vi "atk_def.vi"(9 "IA State":T6, 10 "balls":T7[](array[typedef]), 11 "Robot in":T1) -> (3 "Robot out":T1)   [LabVIEW 2018]
uses:
  Core/AI Robot.ctl
  Functions Enum.ctl
  AttackerStates.ctl
  Path Planning/RRT/PathDests.ctl
  Path Planning/RRT/PathDest.ctl
  Core/AI Ball.ctl
  Core/AI Input.ctl
  Core/Field Size.ctl
  Core/AI Judge.ctl
  Command Enum.ctl
  Util/Events/Events.ctl
  <vilib>/Analysis/_algsub.llb/Real Vector Norm.vi
  <vilib>/Analysis/NI_AALPro.lvlib
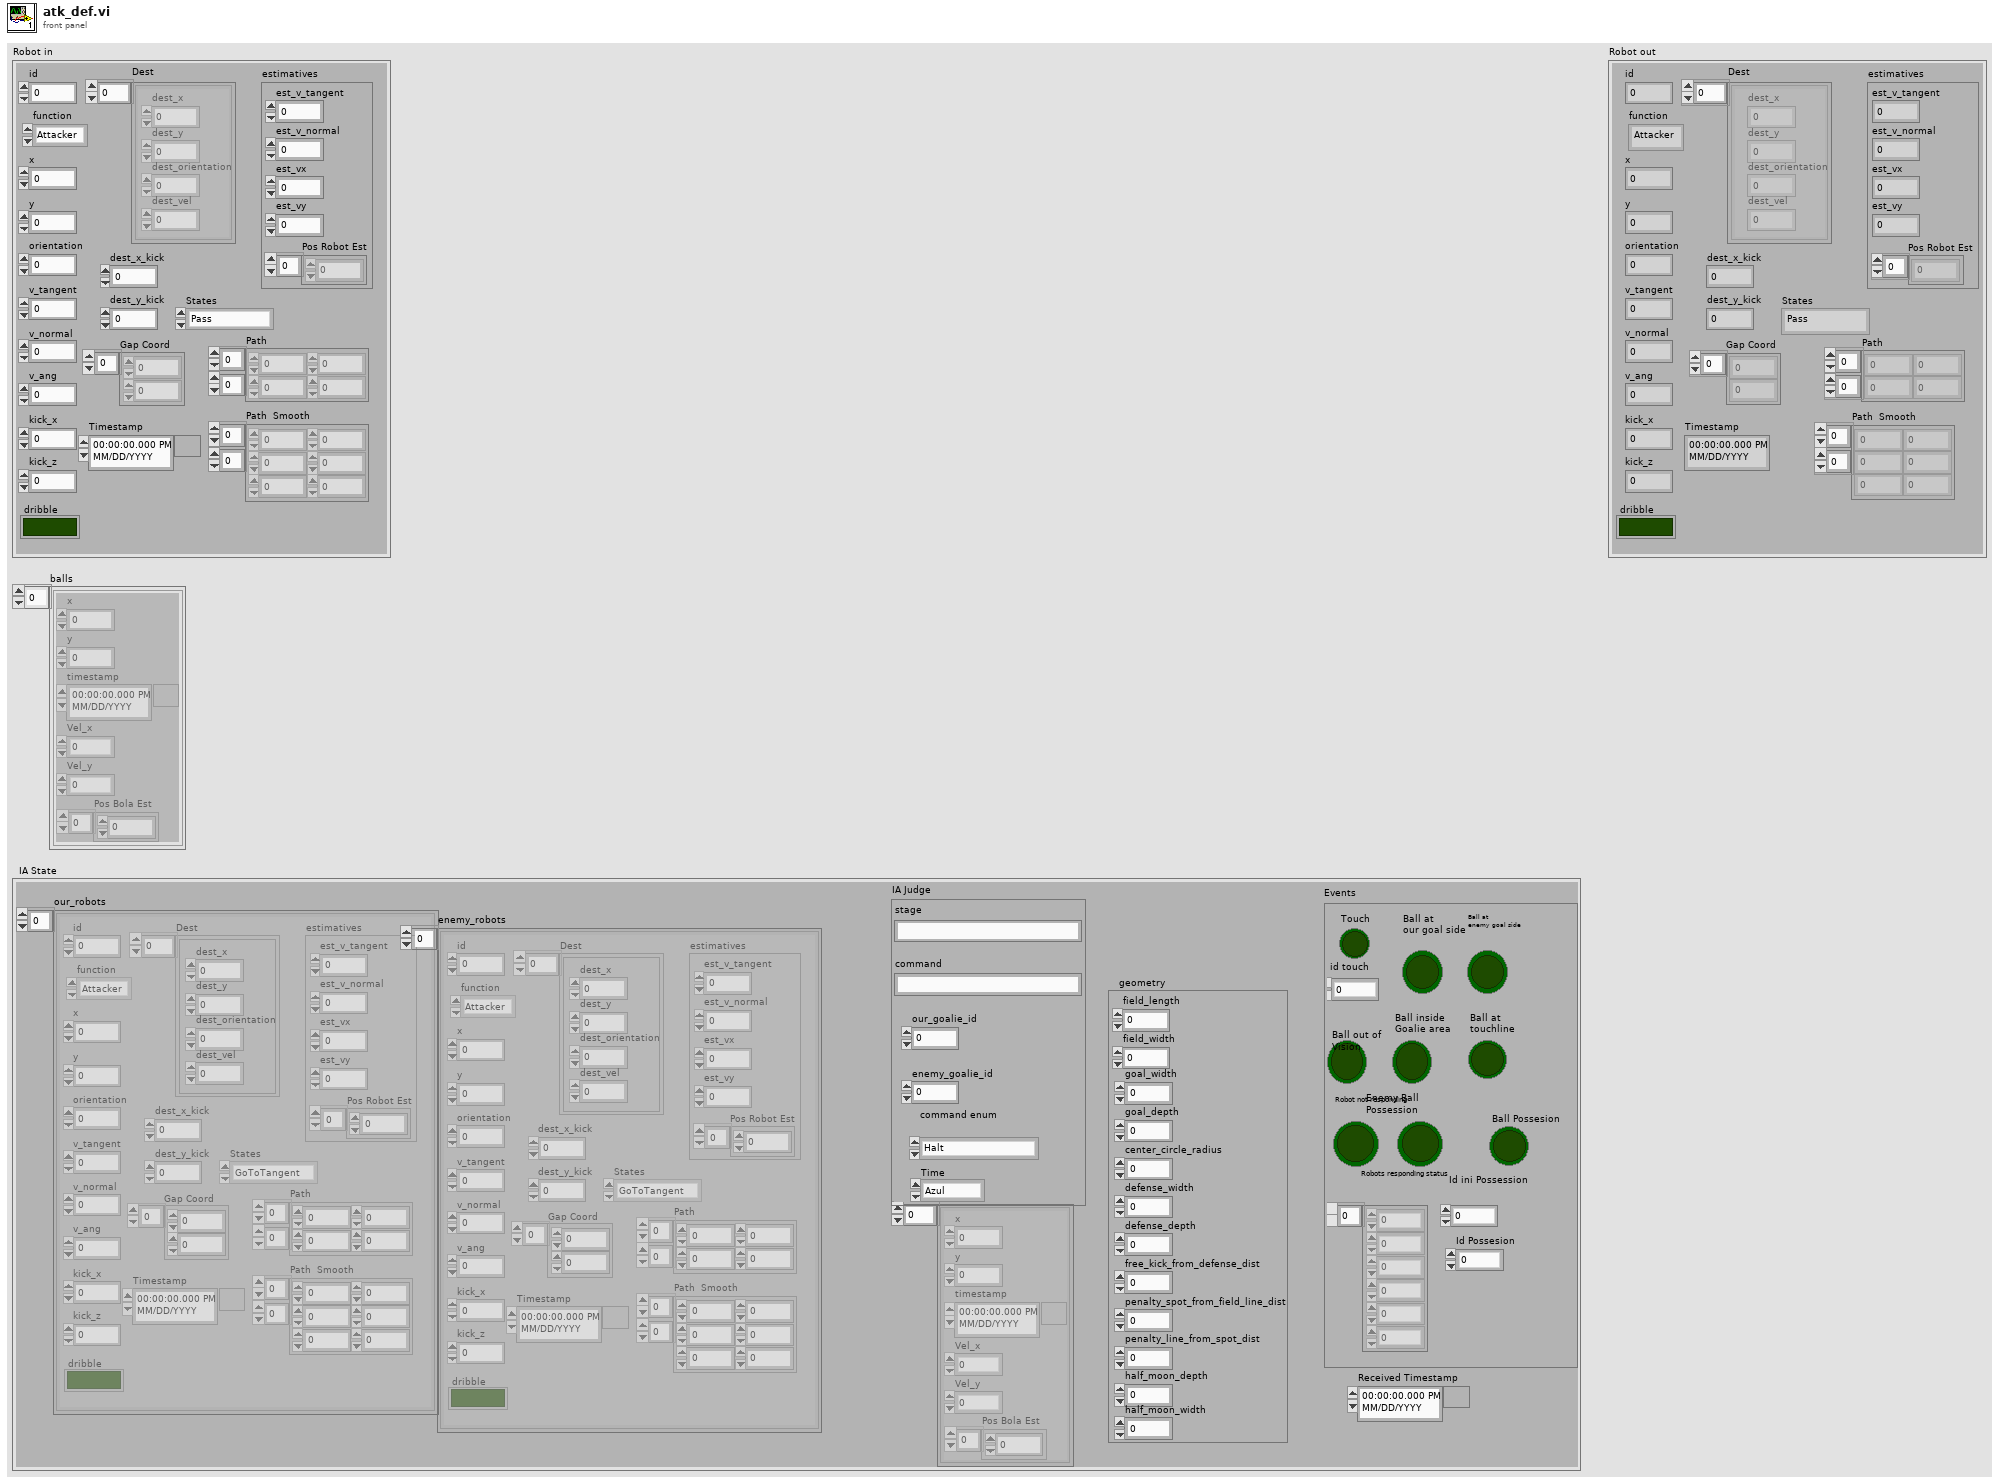
[diagram p1: front panel]
types:
  T1 = typedef "AI Robot.ctl" = cluster{"id":u32, "function":T2, "x":dbl, "y":dbl, "orientation":dbl, "v_tangent":dbl, "v_normal":dbl, "v_ang":dbl, "kick_x":dbl, "kick_z":dbl, "dribble":bool, "Timestamp":timestamp, "estimatives":cluster{"est_v_tangent":dbl, "est_v_normal":dbl, "est_vx":dbl, "est_vy":dbl, "Pos Robot Est":dbl[]}, "dest_x_kick":dbl, "dest_y_kick":dbl, "Gap Coord":dbl[], "States":T3, "Path ":dbl[][], "Path  Smooth":dbl[][], "Dest":T4}
  T2 = typedef "Functions Enum.ctl" = enum16{"Attacker", "Goalie", "Defender", "Striker", "Goto 0", "Dummy", "Kicker", "ZigZag"}
  T3 = typedef "AttackerStates.ctl" = enum16{"Pass", "GoToTangent", "BallGetting", "GoToKick", "Rotate anti-clockwise", "Rotate Clockwise", ""}
  T4 = typedef "PathDests.ctl" = T5[]
  T5 = typedef "PathDest.ctl" = cluster{"dest_x":dbl, "dest_y":dbl, "dest_orientation":dbl, "dest_vel":dbl}
  T6 = typedef "AI Input.ctl" = cluster{"our_robots":T1[], "enemy_robots":T1[], "balls":T7[], "geometry":T8, "IA Judge":T9, "Received Timestamp":timestamp, "Events":T11}
  T7 = typedef "AI Ball.ctl" = cluster{"x":dbl, "y":dbl, "timestamp":timestamp, "Vel_x":dbl, "Vel_y":dbl, "Pos Bola Est":dbl[]}
  T8 = typedef "Field Size.ctl" = cluster{"field_length":u32, "field_width":u32, "goal_width":u32, "goal_depth":u32, "center_circle_radius":u32, "defense_width":u32, "defense_depth":u32, "free_kick_from_defense_dist":u32, "penalty_spot_from_field_line_dist":u32, "penalty_line_from_spot_dist":u32, "half_moon_depth":u32, "half_moon_width":u32}
  T9 = typedef "AI Judge.ctl" = cluster{"stage":string, "command":string, "our_goalie_id":dbl, "enemy_goalie_id":dbl, "command enum":T10, "Time":enum16{"Azul", "Amarelo"}}
  T10 = typedef "Command Enum.ctl" = enum16{"Halt", "Stop", "Force Start", "PKA Normal Start", "Prepare Kickoff Ally", "PKE Normal Start", "Prepare Kickoff Enemy", "Prepare Penalty Ally", "PPA Normal Start", "Prepare Penalty Enemy", "PPE Normal Start", "Ball Placement Enemy Up", "Ball Placement Enemy Down", "Ball Placement Ally Up", "Ball Placement Ally Mid", "Ball Placement Ally Down", "Indirect Free Enemy", "Indirect Free Ally", "Timeout Enemy", "Timeout Ally", "Goal Enemy", "Goal Ally", "Normal Half Time", "Extra Time Break", "Extra Half Time", "None", "Post Game"}
  T11 = typedef "Events.ctl" = cluster{"Touch":bool, "id touch":dbl, "Ball out of \nVision":bool, "Ball inside \nGoalie area":bool, "Robot not responding":bool, "Robots responding status":dbl[], "Enemy Ball \nPossession":bool, "Id ini Possession":dbl, "Ball Possesion":bool, "Id Possesion":dbl, "Ball at\nour goal side":bool, "Ball at\ntouchline":bool, "Ball at\nenemy goal side":bool}
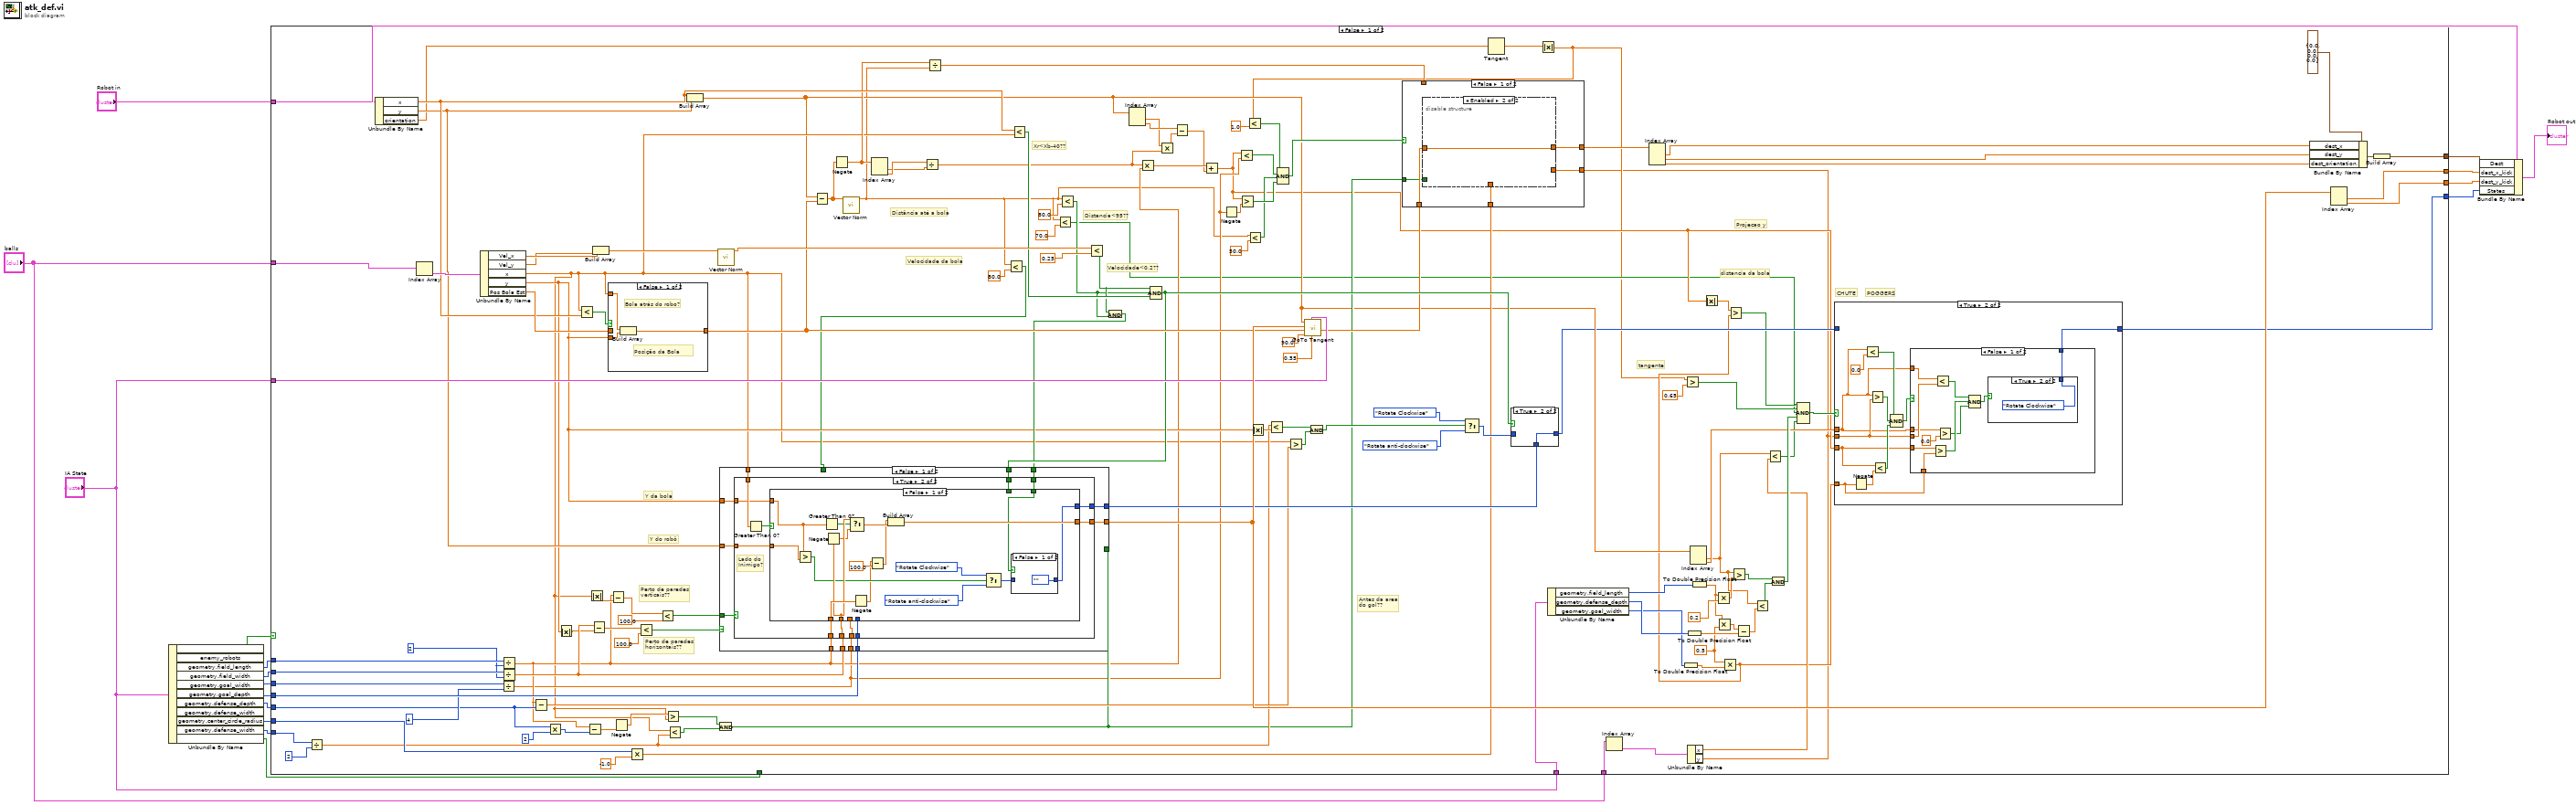
[diagram p0: block diagram]
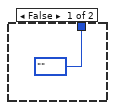
[diagram p3: hidden frame]
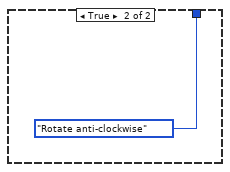
[diagram p4: hidden frame]
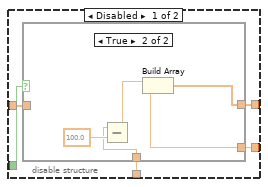
[diagram p5: hidden frame]
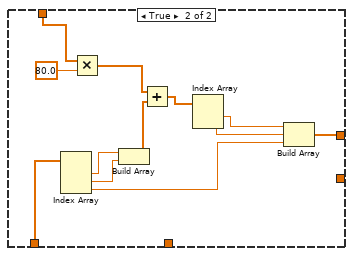
[diagram p7: hidden frame]
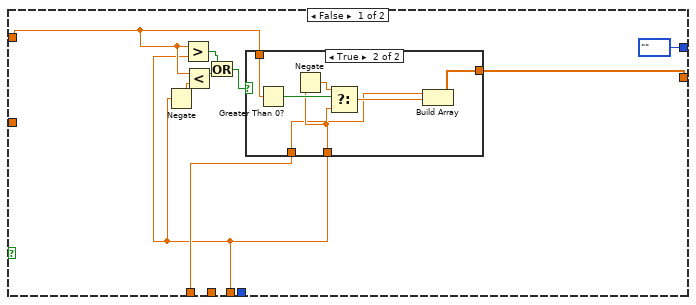
[diagram p10: hidden frame]
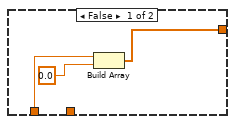
[diagram p11: hidden frame]
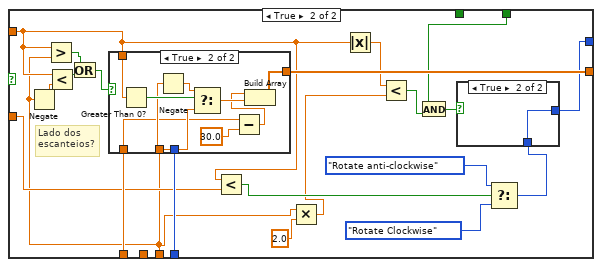
[diagram p13: hidden frame]
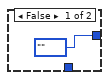
[diagram p14: hidden frame]
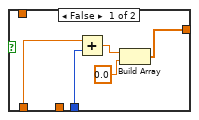
[diagram p15: hidden frame]
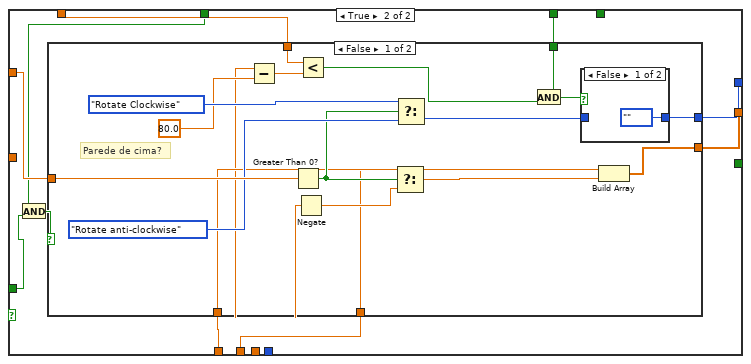
[diagram p16: hidden frame]
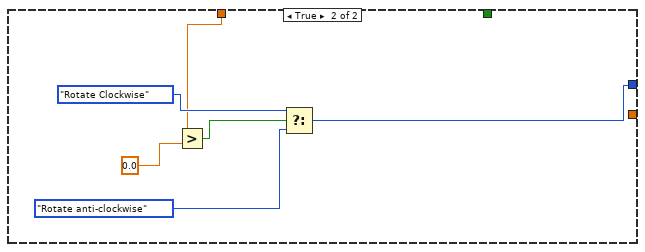
[diagram p18: hidden frame]
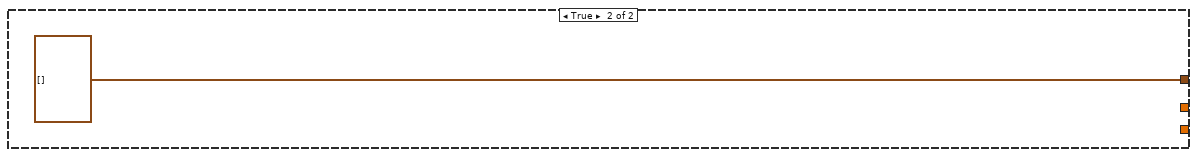
[diagram p19: hidden frame]
diagram:
  n1 = Unbundle By Name("IA State") -> ("Events.Ball out of \nVision"=w12:bool, "geometry.field_length"=w5:u32, "geometry.field_width"=w4:u32, "geometry.goal_width"=w3:u32, "geometry.goal_depth"=w9:u32, "geometry.defense_depth"=w11:u32, "geometry.center_circle_radius"=w14:u32, "geometry.defense_width"=w10:u32, "Events.Ball inside \nGoalie area"=w13:bool)  [unwired: 2 out]
  n2 = case shown="False" w12 {
    tunnel: [w151 _] -> w1
    tunnel: [w150 _] -> w2
    tunnel: w3 -> [w148 _]
    tunnel: "IA State" -> [w147 _]
    tunnel: w4 -> [w143 _]
    tunnel: w5 -> [w142 _]
    tunnel: "Robot in" -> [w141 _]
    tunnel: "balls" -> [w140 _]
    tunnel: [w137 T5[] []] -> w7
    tunnel: w9 -> [w136 _]
    tunnel: w10 -> [w135 _]
    tunnel: w11 -> [w96 _]
    tunnel: w13 -> [_ _]
    tunnel: w14 -> [w90 _]
    tunnel: "IA State" -> [w56 _]
    tunnel: "balls" -> [w58 _]
    tunnel: [w30 _] -> w17
    frame False {
      w36 = 0.5 ("y")
      w130 = u32 2 ("y")
      # "Y do robô"
      # "Y da bola"
      # "distancia da bola"
      # "tangente"
      # "Projecao y"
      # "POGGERS"
      # "CHUTE"
      # "Antes da area \ndo gol??"
      # "Perto de paredes \nverticais??"
      # "Perto de paredes \nhorizontais??"
      # "Velocidade<0,2??"
      # "Distancia<95??"
      # "Xr<Xb-40??"
      # "Velocidade da bola"
      # "Distância até a bola"
      n3 = Divide(x=w135, y=u32 2) -> (x/y=w86:dbl)
      n4 = Unbundle By Name(w141) -> ("x"=w113:dbl, "y"=w100:dbl, "orientation"=w51:dbl)
      n5 = Index Array(array=w140) -> (element=w133:T7)  [unwired: 1 in]
      n6 = Unbundle By Name(w133) -> ("Vel_x"=w123:dbl, "Vel_y"=w122:dbl, "x"=w59:dbl, "y"=w93:dbl, "Pos Bola Est"=w114:dbl[])
      n7 = Divide(x=w148, y=u32 4) -> (x/y=w67:dbl)
      n8 = Divide(x=w142, y=w130) -> (x/y=w75:dbl)
      n9 = Divide(x=w143, y=w130) -> (x/y=w117:dbl)
      n10 = Subtract(x=w75, y=w96) -> (x-y=w104:dbl)
      n11 = Multiply(x=w96, y=u32 2) -> (x*y=w95:u32)
      n12 = Absolute Value(x=w93) -> (abs(x)=w85:dbl)
      n13 = Less?(x=w59, y=w113) -> (x < y?=w116:bool)
      n14 = Subtract(x=w75, y=w95) -> (x-y=w94:dbl)
      n15 = Absolute Value(x=w59) -> (abs(x)=w129:dbl)
      n16 = Subtract(x=w117, y=w85) -> (x-y=w127:dbl)
      n17 = Build Array(w123, w122) -> (w121:dbl[])
      n18 = case shown="False" w116 {
        tunnel: [w209 w212] -> w115
        tunnel: w114 -> [_ w212]
        tunnel: w59 -> [w211 _]
        tunnel: w93 -> [w210 _]
        frame False {
          # "Bola atrás do robo?"
          # "Posição da Bola"
          n19 = Build Array(w211, w210) -> (w209:dbl[])
        }
        frame True {
          # "Posição futura da bola"
          # "Bola atrás do robo?"
        }
      }
      n20 = Subtract(x=w75, y=w129) -> (x-y=w128:dbl)
      n21 = Negate(x=w94) -> (-x=w92:dbl)
      n22 = Multiply(x=w90, y=-1.0) -> (x*y=w87:dbl)
      n23 = Less?(x=w127, y=100.0) -> (x < y?=w126:bool)
      n24 = Less?(x=w128, y=100.0) -> (x < y?=w125:bool)
      n25 = Greater?(x=w92, y=w59) -> (0:w83:bool)
      n26 = Less?(x=w59, y=w86) -> (x < y?=w84:bool)
      n27 = Build Array(w113, w100) -> (w53:dbl[])
      n28 = call-poly <vilib>:"Vector Norm.vi"("Input Vector"=w121) -> ("norm"=w119:dbl)  [unwired: 9 in, 1 out]
      n29 = And(x=w83, y=w84) -> (x .and. y?=w82:bool)
      n30 = Subtract(x=w53, y=w115) -> (x-y=w78:dbl[])
      n31 = Negate(x=w78) -> (-x=w61:dbl[])
      n32 = call-poly <vilib>:"Vector Norm.vi"("Input Vector"=w78) -> ("norm"=w22:dbl)  [unwired: 9 in, 1 out]
      n33 = Index Array(array=w61) -> (element #1=w76:dbl, element #2=w77:dbl)  [unwired: 2 in]
      n34 = Divide(x=w77, y=w76) -> (x/y=w71:dbl)
      n35 = Divide(x=w61, y=w22) -> (x/y=w60:dbl[])
      n36 = Less?(x=w22, y=80.0) -> (x < y?=w79:bool)
      n37 = Less?(x=w113, y=w59) -> (x < y?=w112:bool)
      n38 = Less?(x=w22, y=70.0) -> (x < y?=w23:bool)
      n39 = Less?(x=w22, y=80.0) -> (x < y?=w39:bool)
      n40 = Less?(x=w119, y=0.25) -> (x < y?=w99:bool)
      n41 = And(x=w99, y=w39) -> (x .and. y?=w98:bool)
      n42 = Index Array(array=w53) -> (element #1=w72:dbl, element #2=w74:dbl)  [unwired: 2 in]
      n43 = Multiply(x=w71, y=w75) -> (x*y=w73:dbl)
      n44 = Compound Arithmetic op=AND(w99, w39, w112) -> (w107:bool)
      n45 = case shown="False" w126 {
        tunnel: w93 -> [w222 w321]
        tunnel: w117 -> [w213 w315]
        tunnel: [w221 w320] -> w149
        tunnel: w125 -> [w224 w313]
        tunnel: w59 -> [w223 w317]
        tunnel: w75 -> [w220 w316]
        tunnel: w67 -> [w216 _]
        tunnel: w107 -> [w219 w318]
        tunnel: [w218 w319] -> w106
        tunnel: w136 -> [w217 _]
        tunnel: w100 -> [w215 _]
        tunnel: w98 -> [w214 _]
        tunnel: w82 -> [_ _]
        tunnel: w79 -> [_ w312]
        frame False {
          n46 = case shown="True" w224 {
            tunnel: w223 -> [_ w254]
            tunnel: w222 -> [w231 w253]
            tunnel: [w232 w252] -> w221
            tunnel: w220 -> [w233 w251]
            tunnel: w219 -> [_ w250]
            tunnel: [AttackerStates."" ("States") w249] -> w218
            tunnel: w217 -> [_ w248]
            tunnel: w213 -> [_ w247]
            tunnel: w216 -> [w229 w246]
            tunnel: w215 -> [_ w245]
            tunnel: w214 -> [_ w244]
            frame False {
              n47 = Negate(x=w229) -> (-x=w228:dbl)
              n48 = Greater?(x=w231, y=w229) -> (0:w225:bool)
              n49 = Less?(x=w231, y=w228) -> (x < y?=w226:bool)
              n50 = Or(x=w225, y=w226) -> (x .or. y?=w227:bool)
              n51 = case shown="True" w227 {
                tunnel: w233 -> [w235 w238]
                tunnel: [w236 w237] -> w232
                tunnel: w231 -> [_ w242]
                tunnel: w229 -> [_ w240]
                frame False {
                  n52 = Build Array(w235, 0.0 ("element")) -> (w236:dbl[])
                }
                frame True {
                  n53 = Greater Than 0?(x=w242) -> (x > 0?=w243:bool)
                  n54 = Negate(x=w240) -> (-x=w241:dbl)
                  n55 = Select(t=w241, s=w243, f=w240) -> (s? t:f=w239:dbl)
                  n56 = Build Array(w238, w239) -> (w237:dbl[])
                }
              }
            }
            frame True {
              # "Lado do\nInimigo?"
              n57 = Greater Than 0?(x=w254) -> (x > 0?=w255:bool)
              n58 = case shown="False" w255 {
                tunnel: w253 -> [w268 w286]
                tunnel: [w272 w290] -> w252
                tunnel: w251 -> [w270 w291]
                tunnel: w250 -> [_ _]
                tunnel: [w271 w281] -> w249
                tunnel: w248 -> [_ w289]
                tunnel: w247 -> [w269 _]
                tunnel: w246 -> [_ w276]
                tunnel: w245 -> [w267 w285]
                tunnel: w244 -> [w266 w278]
                frame False {
                  n59 = Greater?(x=w268, y=w267) -> (0:w259:bool)
                  n60 = Greater Than 0?(x=w268) -> (x > 0?=w262:bool)
                  n61 = Negate(x=w269) -> (-x=w265:dbl)
                  n62 = Select(t=w269, s=w262, f=w265) -> (s? t:f=w264:dbl)
                  n63 = Negate(x=w270) -> (-x=w256:dbl)
                  n64 = Subtract(x=w256, y=100.0) -> (x-y=w257:dbl)
                  n65 = Build Array(w257, w264) -> (w272:dbl[])
                  n66 = Select(t=AttackerStates."Rotate Clockwise" ("States"), s=w259, f=AttackerStates."Rotate anti-clockwise" ("States")) -> (s? t:f=w260:T3)
                  n67 = case shown="False" w266 {
                    tunnel: [AttackerStates."" ("States") w274] -> w271
                    tunnel: w260 -> [_ w274]
                    frame False {
                    }
                    frame True {
                    }
                  }
                }
                frame True {
                  # "Lado dos\nescanteios?"
                  n68 = Negate(x=w276) -> (-x=w295:dbl)
                  n69 = Greater?(x=w286, y=w276) -> (0:w292:bool)
                  n70 = Less?(x=w286, y=w295) -> (x < y?=w293:bool)
                  n71 = Or(x=w292, y=w293) -> (x .or. y?=w294:bool)
                  n72 = case shown="True" w294 {
                    tunnel: w291 -> [w298 w303]
                    tunnel: [w301 w306] -> w290
                    tunnel: w286 -> [_ w310]
                    tunnel: w276 -> [_ w308]
                    tunnel: w289 -> [w299 _]
                    frame False {
                      n73 = Add(x=w298, y=w299) -> (x+y=w300:dbl)
                      n74 = Build Array(w300, 0.0 ("element")) -> (w301:dbl[])
                    }
                    frame True {
                      n75 = Greater Than 0?(x=w310) -> (x > 0?=w311:bool)
                      n76 = Negate(x=w308) -> (-x=w309:dbl)
                      n77 = Select(t=w309, s=w311, f=w308) -> (s? t:f=w307:dbl)
                      n78 = Subtract(x=w303, y=30.0) -> (x-y=w304:dbl)
                      n79 = Build Array(w304, w307) -> (w306:dbl[])
                    }
                  }
                  n80 = Less?(x=w286, y=w285) -> (x < y?=w284:bool)
                  n81 = Multiply(x=w276, y=2.0) -> (x*y=w275:dbl)
                  n82 = Absolute Value(x=w286) -> (abs(x)=w288:dbl)
                  n83 = Less?(x=w288, y=w275) -> (x < y?=w279:bool)
                  n84 = And(x=w278, y=w279) -> (x .and. y?=w280:bool)
                  n85 = Select(t=AttackerStates."Rotate anti-clockwise" ("States"), s=w284, f=AttackerStates."Rotate Clockwise" ("States")) -> (s? t:f=w287:T3)
                  n86 = case shown="True" w280 {
                    tunnel: w287 -> [_ w297]
                    tunnel: [AttackerStates."" ("States") w297] -> w281
                    frame False {
                    }
                    frame True {
                    }
                  }
                }
              }
            }
          }
        }
        frame True {
          n87 = And(x=w312, y=w313) -> (x .and. y?=w314:bool)
          n88 = case shown="False" w314 {
            tunnel: w321 -> [w338 _]
            tunnel: [w335 _] -> w320
            tunnel: [w332 w341] -> w319
            tunnel: w318 -> [w330 _]
            tunnel: w317 -> [w329 w342]
            tunnel: w316 -> [w323 _]
            tunnel: w315 -> [w322 _]
            frame False {
              # "Parede de cima?"
              n89 = Subtract(x=w322, y=80.0) -> (x-y=w328:dbl)
              n90 = Greater Than 0?(x=w338) -> (x > 0?=w331:bool)
              n91 = Negate(x=w322) -> (-x=w337:dbl)
              n92 = Less?(x=w329, y=w328) -> (x < y?=w325:bool)
              n93 = Select(t=w322, s=w331, f=w337) -> (s? t:f=w336:dbl)
              n94 = Select(t=AttackerStates."Rotate Clockwise" ("States"), s=w331, f=AttackerStates."Rotate anti-clockwise" ("States")) -> (s? t:f=w326:T3)
              n95 = And(x=w330, y=w325) -> (x .and. y?=w324:bool)
              n96 = case shown="False" w324 {
                tunnel: w326 -> [_ w340]
                tunnel: [AttackerStates."" ("States") w340] -> w332
                frame False {
                }
                frame True {
                }
              }
              n97 = Build Array(w323, w336) -> (w335:dbl[])
            }
            frame True {
              n98 = Greater?(x=w342, y=0.0) -> (0:w343:bool)
              n99 = Select(t=AttackerStates."Rotate Clockwise" ("States"), s=w343, f=AttackerStates."Rotate anti-clockwise" ("States")) -> (s? t:f=w341:T3)
            }
          }
        }
      }
      n100 = Multiply(x=w72, y=w71) -> (x*y=w70:dbl)
      n101 = Subtract(x=w74, y=w70) -> (x-y=w69:dbl)
      n102 = Add(x=w73, y=w69) -> (x+y=w28:dbl)
      n103 = Negate(x=w67) -> (-x=w68:dbl)
      n104 = Less?(x=w28, y=w67) -> (x < y?=w66:bool)
      n105 = Greater?(x=w28, y=w68) -> (0:w65:bool)
      n106 = Less?(x=w22, y=50.0) -> (x < y?=w63:bool)
      n107 = Absolute Value(x=w93) -> (abs(x)=w105:dbl)
      n108 = Less?(x=w86, y=w105) -> (x < y?=w103:bool)
      n109 = Greater?(x=w59, y=w104) -> (0:w102:bool)
      n110 = call "GoTo Tangent.vi"("Cone de chute"=0.55, "IA State Input in"=w147, "distance between ball and robot"=90.0, "Ball"=w115, "Target"=w149, "R"=w53) -> ("Destination"=w89:dbl[])  [unwired: 4 in, 1 out]
      n111 = And(x=w103, y=w102) -> (x .and. y?=w101:bool)
      n112 = Select(t=AttackerStates."Rotate Clockwise" ("States"), s=w101, f=AttackerStates."Rotate anti-clockwise" ("States")) -> (s? t:f=w108:T3)
      n113 = Tangent(1:w51) -> (0:w50:dbl)
      n114 = case shown="True" w107 {
        tunnel: [w207 w208] -> w31
        tunnel: w108 -> [_ _]
        tunnel: w106 -> [w207 w208]
        frame False {
        }
        frame True {
        }
      }
      n115 = Absolute Value(x=w50) -> (abs(x)=w21:dbl)
      n116 = Less?(x=w21, y=1.0) -> (x < y?=w19:bool)
      n117 = Compound Arithmetic op=AND(w19, w66, w63, w65) -> (w62:bool)
      n118 = Unbundle By Name(w56) -> ("geometry.field_length"=w54:u32, "geometry.defense_depth"=w46:u32, "geometry.goal_width"=w37:u32)
      n119 = Index Array(array=w58) -> (element=w57:T7)  [unwired: 1 in]
      n120 = To Double Precision Float(number=w37) -> (double precision float=w27:dbl)
      n121 = Greater?(x=w21, y=0.65) -> (0:w48:bool)
      n122 = To Double Precision Float(number=w46) -> (double precision float=w45:dbl)
      n123 = Unbundle By Name(w57) -> ("x"=w33:dbl, "y"=w18:dbl)
      n124 = case shown="False" w62 {
        tunnel: w89 -> [w182 w206]
        tunnel: [w181 w195] -> w88
        tunnel: w87 -> [w180 _]
        tunnel: w82 -> [w179 _]
        tunnel: w60 -> [_ w204]
        tunnel: w18 -> [w178 _]
        frame False {
          n125 = disable-structure shown="Enabled" {
            disable-tunnel: w182 -> [w187 w194]
            disable-tunnel: [w186 w194] -> w181
            disable-tunnel: w180 -> [w185 _]
            disable-tunnel: w179 -> [w184 _]
            disable-tunnel: w178 -> [w183 _]
            frame Disabled {
              n126 = case shown="True" w184 {
                tunnel: [w188 w193] -> w186
                tunnel: w187 -> [w188 _]
                tunnel: w185 -> [_ w190]
                tunnel: w183 -> [_ w189]
                frame False {
                }
                frame True {
                  n127 = Subtract(x=w190, y=100.0) -> (x-y=w191:dbl)
                  n128 = Build Array(w191, w189) -> (w193:dbl[])
                }
              }
            }
            frame Enabled {
            }
          }
        }
        frame True {
          n129 = Index Array(array=w206) -> (element #1=w201:dbl, element #2=w200:dbl, element #3=w196:dbl)  [unwired: 3 in]
          n130 = Multiply(x=w204, y=80.0) -> (x*y=w203:dbl[])
          n131 = Build Array(w201, w200) -> (w202:dbl[])
          n132 = Add(x=w203, y=w202) -> (x+y=w199:dbl[])
          n133 = Index Array(array=w199) -> (element #1=w198:dbl, element #2=w197:dbl)  [unwired: 2 in]
          n134 = Build Array(w198, w197, w196) -> (w195:dbl[])
        }
      }
      n135 = Index Array(array=w88) -> (element #1=w145:dbl, element #2=w146:dbl, element #3=w144:dbl)  [unwired: 3 in]
      n136 = Index Array(array=w53) -> (element #1=w32:dbl, element #2=w35:dbl)  [unwired: 2 in]
      n137 = To Double Precision Float(number=w54) -> (double precision float=w47:dbl)
      n138 = Absolute Value(x=w28) -> (abs(x)=w29:dbl)
      n139 = Multiply(x=w47, y=0.2) -> (x*y=w52:dbl)
      n140 = Multiply(x=w47, y=w36) -> (x*y=w44:dbl)
      n141 = Multiply(x=w36, y=w27) -> (x*y=w25:dbl)
      n142 = Greater?(x=w29, y=w25) -> (0:w26:bool)
      n143 = Greater?(x=w32, y=w52) -> (0:w41:bool)
      n144 = Subtract(x=w44, y=w45) -> (x-y=w43:dbl)
      n145 = Less?(x=w32, y=w43) -> (x < y?=w42:bool)
      n146 = Less?(x=w32, y=w33) -> (x < y?=w34:bool)
      n147 = And(x=w41, y=w42) -> (x .and. y?=w40:bool)
      n148 = Compound Arithmetic op=AND(w26, w48, w23, w40, w34) -> (w38:bool)
      n149 = case shown="True" w38 {
        tunnel: w28 -> [_ w153]
        tunnel: w35 -> [_ w155]
        tunnel: w25 -> [_ w160]
        tunnel: w18 -> [_ w159]
        tunnel: w31 -> [w152 _]
        tunnel: [w152 w158] -> w30
        frame False {
        }
        frame True {
          n150 = Negate(x=w160) -> (-x=w154:dbl)
          n151 = Less?(x=w155, y=0.0) -> (x < y?=w156:bool)
          n152 = Greater?(x=w155, y=w159) -> (0:w162:bool)
          n153 = Less?(x=w153, y=w154) -> (x < y?=w163:bool)
          n154 = Compound Arithmetic op=AND(w156, w162, w163) -> (w161:bool)
          n155 = case shown="False" w161 {
            tunnel: w160 -> [w169 _]
            tunnel: w153 -> [w170 _]
            tunnel: w159 -> [w171 _]
            tunnel: w155 -> [w174 _]
            tunnel: [w167 AttackerStates."Rotate anti-clockwise" ("States")] -> w158
            tunnel: w155 -> [w165 _]
            frame False {
              n156 = Greater?(x=w170, y=w169) -> (0:w172:bool)
              n157 = Less?(x=w174, y=w171) -> (x < y?=w173:bool)
              n158 = Greater?(x=w165, y=0.0) -> (0:w164:bool)
              n159 = Compound Arithmetic op=AND(w173, w172, w164) -> (w168:bool)
              n160 = case shown="True" w168 {
                tunnel: [AttackerStates."" ("States") AttackerStates."Rotate Clockwise" ("States")] -> w167
                frame False {
                }
                frame True {
                }
              }
            }
            frame True {
            }
          }
        }
      }
      n161 = Bundle By Name(cluster=T5 {"dest_x"=0.0, "dest_y"=0.0, "dest_orientation"=0.0, "dest_vel"=0.0} ("element"), "dest_x"=w145, "dest_y"=w146, "dest_orientation"=w144) -> (w138:T5)
      n162 = Index Array(array=w149) -> (element #1=w150:dbl, element #2=w151:dbl)  [unwired: 2 in]
      n163 = Build Array(w138) -> (w137:T5[])
    }
    frame True {
    }
  }
  n164 = Bundle By Name(cluster="Robot in", "Dest"=w7, "dest_x_kick"=w2, "dest_y_kick"=w1, "States"=w17) -> (→"Robot out":T1)
